vi "Warning Fault Tree View.vi"(0 "Model in":refnum<class "Model.lvclass">) -> ()   [LabVIEW 2016, in "M1M3SupportEUI_Views.lvlib"]
uses:
  M1M3SupportEUI_Views.lvlib
  Model/Model.lvclass
  M1M3 Support Events/M1M3 Support Events.lvclass/M1M3 Support Events.ctl
  M1M3 Support Events/M1M3 Support Events.lvclass
  EUI Events/EUI Events.lvclass
panel:
  in  "ClearAllErrors":bool
  in  "ClearOneError":bool
  in  "WarningTree":string(tree)
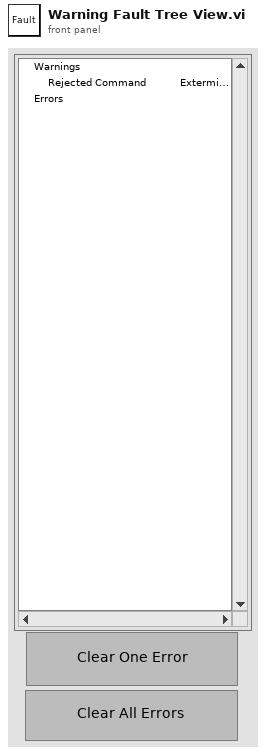
[diagram p1: front panel]
types:
  T1 = typedef "M1M3SupportEUI_TypeDefs.lvlib/M1M3 Support Events.ctl" = cluster{"Inclinometer  Data":refnum<user-event>, "IMS Data":refnum<user-event>, "SAL Connected":refnum<user-event>, "Accelerometer Data":refnum<user-event>, "OuterLoop Data":refnum<user-event>, "ErrorCode Event":refnum<user-event>, "InterlockStatus Event":refnum<user-event>, "InterlockWarning Event":refnum<user-event>, "Gyro Data":refnum<user-event>, "HP Actuator Info Event":refnum<user-event>, " FA Info Event":refnum<user-event>, "HP Monitor Info Event":refnum<user-event>, "FA Data":refnum<user-event>, "HP Actuator data":refnum<user-event>, "HP Monitor data":refnum<user-event>, "Air Supply Status Event":refnum<user-event>, "Air Supply Warning Event":refnum<user-event>, "Power Data":refnum<user-event>, "PID Data":refnum<user-event>, "PID Info Event":refnum<user-event>, "Power Status Event":refnum<user-event>, "Power Supply Status Event":refnum<user-event>, "Power Warning Event":refnum<user-event>, "Summary State Event":refnum<user-event>, "Detailed State Event":refnum<user-event>, "FA Force Warning Event":refnum<user-event>, "FA Warning Event":refnum<user-event>, "FA State Event":refnum<user-event>, "Applied AberrationForces Event":refnum<user-event>, "Applied Acceleration Forcces Event":refnum<user-event>, "Applied Azimuth Forces Event":refnum<user-event>, "Applied Active Optic Forces Event":refnum<user-event>, "Applied Balance Forces Event":refnum<user-event>, "Applied Cylinder Forces Event":refnum<user-event>, "Applied Elevation Forces Event":refnum<user-event>, "Applied Forces Event":refnum<user-event>, "Applied Offset Forces Event":refnum<user-event>, "Applied Static Forces Event":refnum<user-event>, "Applied Thermal Forces Event":refnum<user-event>, "Applied Velocity Forces Event":refnum<user-event>, "Rejected Aberration Force Event":refnum<user-event>, "Rejected Acceleration Forces Event":refnum<user-event>, "Rejected Active Optic Forces Event":refnum<user-event>, "Rejected Azimuth Forces Event":refnum<user-event>, "Rejected Balance Forces Event":refnum<user-event>, "Rejected Cylinder Forces Event":refnum<user-event>, "Rejected Elevation Forces Event":refnum<user-event>, "Rejected Forces Event":refnum<user-event>, "Rejected Offset Forces Event":refnum<user-event>, "Rejected Static Forces Event":refnum<user-event>, "Rejected Thermal Forces Event":refnum<user-event>, "Rejected Velocity Forces Event":refnum<user-event>, "Command Rejection Event":refnum<user-event>, "Setting Verions Event":refnum<user-event>, "Settings Applied Event":refnum<user-event>, "HP Actuator State Event":refnum<user-event>, "HP Actuator Warning Event":refnum<user-event>, "HP Monitor State Event":refnum<user-event>, "HP Monitor Warning Event":refnum<user-event>, "Accelerometer Warning Event":refnum<user-event>, "Applied Settings Match Start Event":refnum<user-event>, "Cell Light Status Event ":refnum<user-event>, "Cell Light Warning Event":refnum<user-event>, "Displacement Sensor Warning Event":refnum<user-event>, "Force Setpoint Warning Event":refnum<user-event>, "Gyro Warning Event ":refnum<user-event>, "ILC Warning Event ":refnum<user-event>, "Inclinometer Sensor Warning Event ":refnum<user-event>}
  T2 = enum16{"", "DetailedState_DetailedStates_DisabledState", "DetailedState_DetailedStates_EnabledState", "DetailedState_DetailedStates_FaultState", "DetailedState_DetailedStates_OfflineState", "DetailedState_DetailedStates_StandbyState", "DetailedState_DetailedStates_ParkedState", "DetailedState_DetailedStates_RaisingState", "DetailedState_DetailedStates_ActiveState", "DetailedState_DetailedStates_LoweringState", "DetailedState_DetailedStates_EngineeringState", "DetailedState_DetailedStates_ParkedEngineeringState", "DetailedState_DetailedStates_RaisingEngineeringState", "DetailedState_DetailedStates_ActiveEngineeringState", "DetailedState_DetailedStates_LoweringEngineeringState", "DetailedState_DetailedStates_LoweringFaultState", "DetailedState_DetailedStates_ProfileHardpointCorrectionState"}
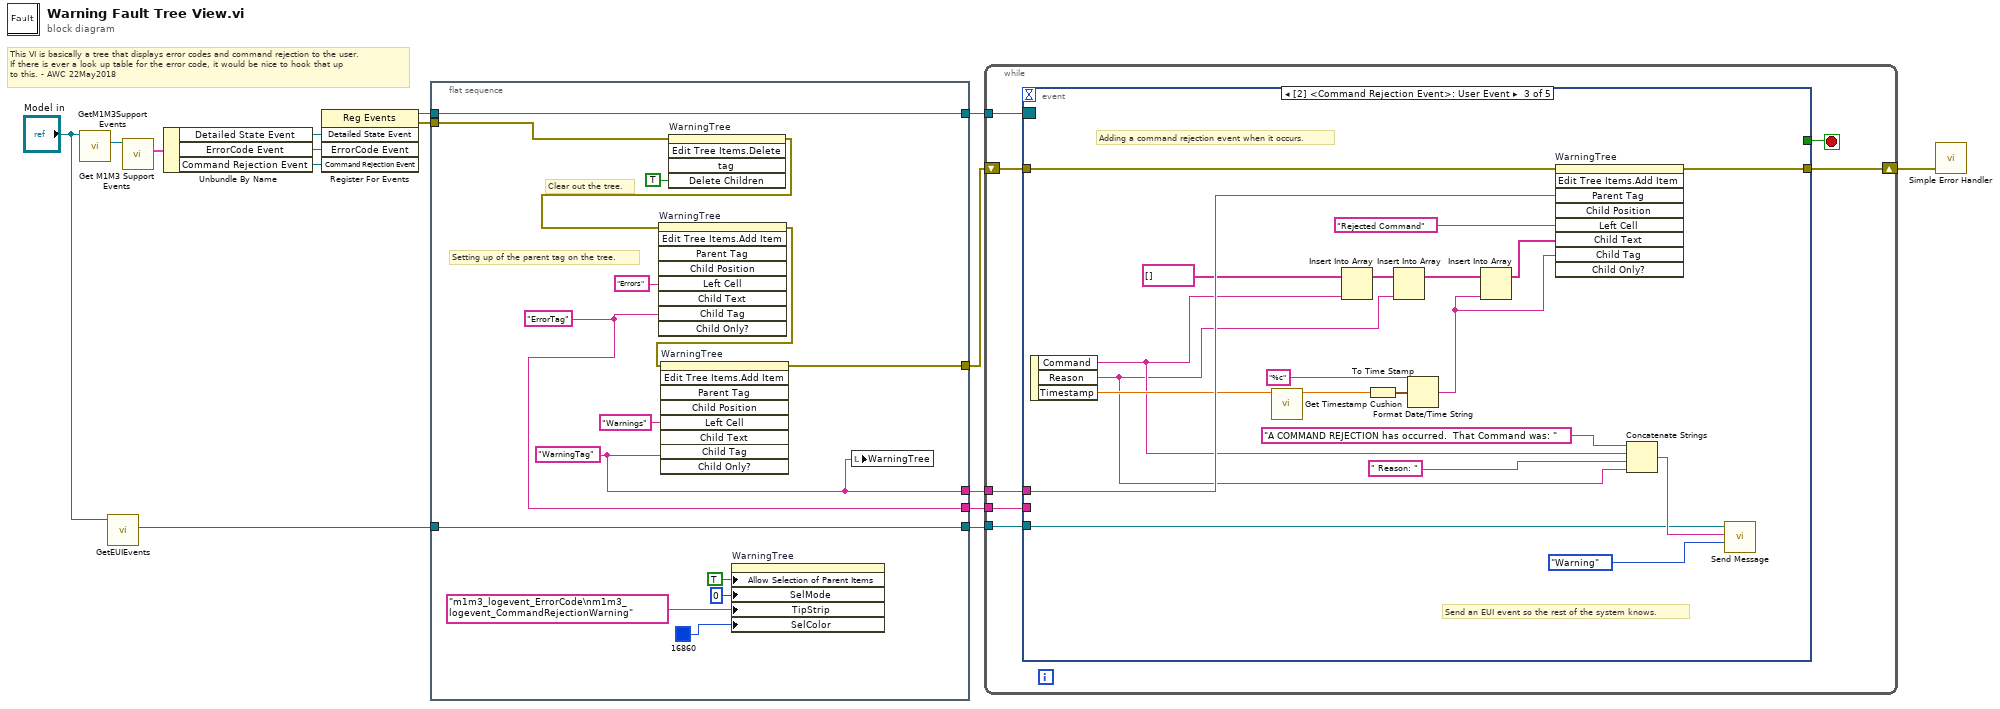
[diagram p0: block diagram]
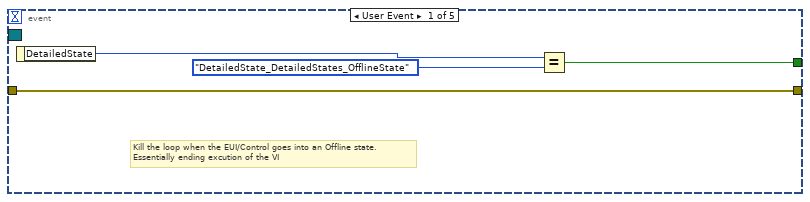
[diagram p2: hidden frame]
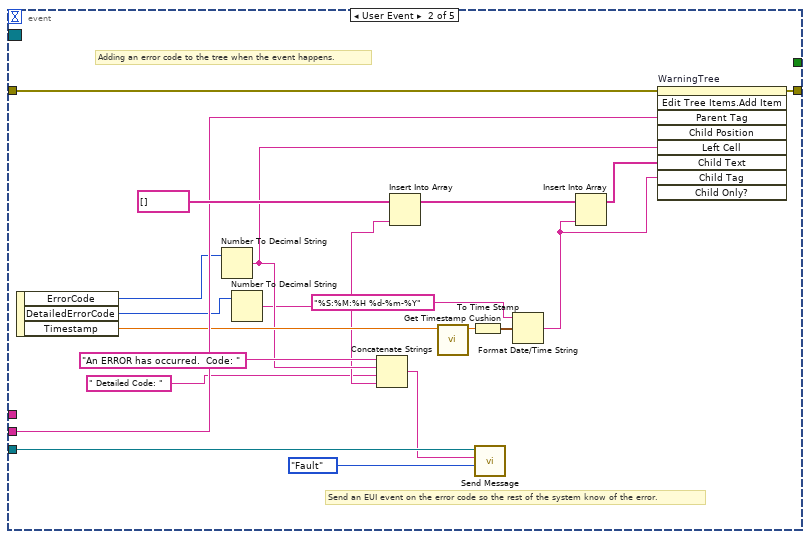
[diagram p3: hidden frame]
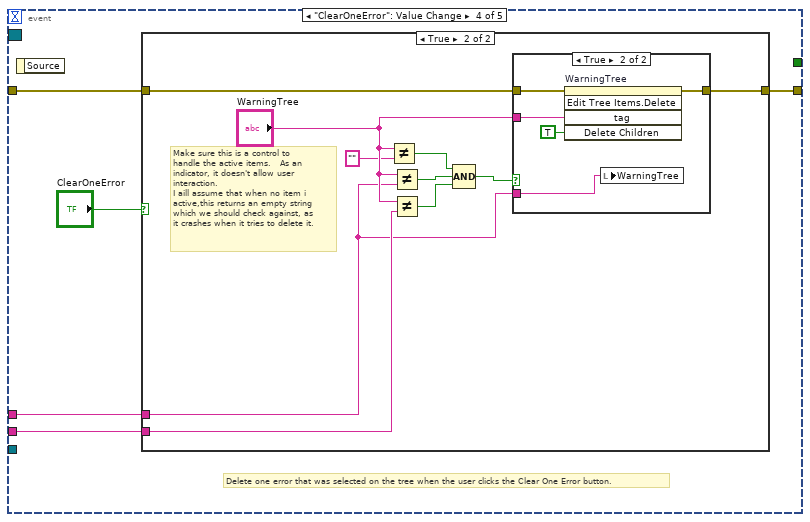
[diagram p4: hidden frame]
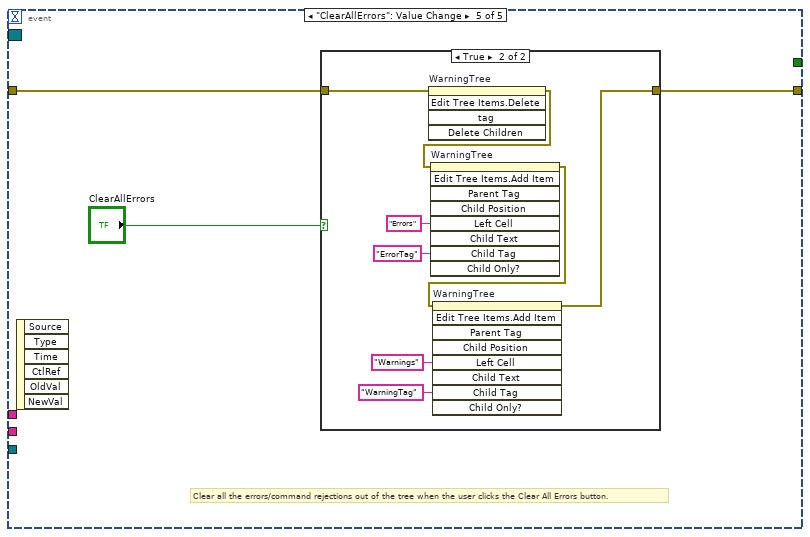
[diagram p7: hidden frame]
diagram:
  # "This VI is basically a tree that displays error codes and command rejection to the user.\nIf there is ever a look up table for the error code, it would be nice to hook that up\nto this. - AWC 22May2018"
  n1 = call "GetM1M3SupportEvents.vi"("Model in"="Model in") -> ("M1M3 Support Events out"=w11:refnum<class "M1M3 Support Events.lvclass">)  [unwired: 8 in, 2 out]
  n2 = call "GetEUIEvents.vi"("Model in"="Model in") -> ("EUI Events out"=w1:refnum<class "EUI Events.lvclass">)  [unwired: 8 in, 2 out]
  n3 = call "Get M1M3 Support Events.vi"("M1M3 Support Events in"=w11) -> ("M1M3 Support Events"=w12:T1)  [unwired: 9 in, 1 out]
  n4 = Unbundle By Name(w12) -> ("Detailed State Event"=w13:refnum<user-event>, "ErrorCode Event"=w14:refnum<user-event>, "Command Rejection Event"=w15:refnum<user-event>)
  n5 = register-events(w13, w14, w15) -> (reference out=w10:refnum<event-registration>, error out=w8:errorcluster)  [unwired: 2 in]
  n6 = flat-sequence {
    tunnel: w10 -> [w30]
    tunnel: [w30] -> w9
    tunnel: w8 -> [w18]
    tunnel: [w17] -> w7
    tunnel: [w16] -> w6
    tunnel: [w25] -> w5
    tunnel: w1 -> [w22]
    tunnel: [w22] -> w2
    frame #0 {
      w16 = "WarningTag" ("Child Tag")
      w25 = "ErrorTag" ("Child Tag")
      # "Clear out the tree."
      # "Setting up of the parent tag on the tree."
      n7 = invoke on="WarningTree" class="Tree (strict)" method="Edit Tree Items.Delete"(error in=w18, "Delete Children"=TRUE ("Delete Children?")) -> (error out=w29:errorcluster)  [unwired: 3 in, 4 out]
      n8 = invoke on="WarningTree" class="Tree (strict)" method="Edit Tree Items.Add Item"(error in=w29, "Left Cell"="Errors" ("Left Cell String"), "Child Tag"=w25) -> (error out=w27:errorcluster)  [unwired: 6 in, 8 out]
      n9 = invoke on="WarningTree" class="Tree (strict)" method="Edit Tree Items.Add Item"(error in=w27, "Left Cell"="Warnings" ("Left Cell String"), "Child Tag"=w16) -> (error out=w17:errorcluster)  [unwired: 6 in, 8 out]
      n10 = property on="WarningTree" class="Tree (strict)"("Allow Selection of Parent Items"=TRUE, "SelMode"=0 ("Selection Mode"), "TipStrip"="m1m3_logevent_ErrorCode\nm1m3_logevent_CommandRejectionWarning" ("Tip Strip"), "SelColor"=u32 16860) -> ()  [unwired: 2 in, 2 out]
      n11 = local write "WarningTree"(w16) -> ()
    }
  }
  n12 = while {
    tunnel: w9 -> [w37]
    shift-right: [w32] -> w4
    shift-left: w7 -> [w35]
    tunnel: w6 -> [w34]
    tunnel: w5 -> [w33]
    tunnel: w2 -> [w31]
    stop <- w36 stop-if-true
    n13 = event shown="[2] <Command Rejection Event>: User Event" {
      selector: w37 -> [_ _ _ _ _]
      dyn-events: _ -> [_ _ _ _ _]
      timeout: _ -> [_ _ _ _ _]
      tunnel: [w39 _ _ _ _] -> w36
      tunnel: w35 -> [w38 w56 w81 w85 w105]
      tunnel: w34 -> [_ _ w80 w83 _]
      tunnel: w33 -> [_ w55 _ w82 _]
      tunnel: [w38 w51 w70 w84 w104] -> w32
      tunnel: w31 -> [_ w49 w66 _ _]
      event User Event {
        # "Kill the loop when the EUI/Control goes into an Offline state.\nEssentially ending excution of the VI"
        n14 = event-data() -> ("DetailedState"=w41:T2)  [unwired: 1 in]
        n15 = Equal?(x=w41, y=T2."DetailedState_DetailedStates_OfflineState") -> (x = y?=w39:bool)
      }
      event User Event {
        # "Send an EUI event on the error code so the rest of the system know of the error."
        # "Adding an error code to the tree when the event happens."
        n16 = event-data() -> ("ErrorCode"=w53:i32, "DetailedErrorCode"=w52:i32, "Timestamp"=w54:dbl)  [unwired: 1 in]
        n17 = Number To Decimal String(number=w53) -> (decimal integer string=w47:string)  [unwired: 1 in]
        n18 = Number To Decimal String(number=w52) -> (decimal integer string=w46:string)  [unwired: 1 in]
        n19 = Concatenate Strings("An ERROR has occurred.  Code: " ("string"), w47, " Detailed Code: " ("string"), w46) -> (w44:string)
        n20 = Insert Into Array(array=string[] [], new element=w46) -> (w60:string[])  [unwired: 1 in]
        n21 = call "Get Timestamp Cushion.vi"("DoubleTimestampRepresentation"=w54) -> ("TimestampCushion"=w58:dbl)  [unwired: 10 in]
        n22 = To Time Stamp(1:w58) -> (0:w57:timestamp)
        n23 = call "Send Message.vi"("Priority"=enum16{"Message", "Warning", "Fault", ""}."Fault", "Message"=w44, "EUI Events in"=w49) -> ()  [unwired: 7 in, 2 out]
        n24 = Format Date/Time String(time format string (%c)="%S:%M:%H %d-%m-%Y", seconds (now)=w57) -> (date/time string=w42:string)  [unwired: 1 in]
        n25 = Insert Into Array(array=w60, new element=w42) -> (w59:string[])  [unwired: 1 in]
        n26 = invoke on="WarningTree" class="Tree (strict)" method="Edit Tree Items.Add Item"(error in=w56, "Parent Tag"=w55, "Left Cell"=w47, "Child Text"=w59, "Child Tag"=w42) -> (error out=w51:errorcluster)  [unwired: 4 in, 8 out]
      }
      event User Event {
        # "Send an EUI event so the rest of the system knows."
        # "Adding a command rejection event when it occurs."
        n27 = event-data() -> ("Command"=w65:string, "Reason"=w64:string, "Timestamp"=w72:dbl)  [unwired: 1 in]
        n28 = call "Get Timestamp Cushion.vi"("DoubleTimestampRepresentation"=w72) -> ("TimestampCushion"=w74:dbl)  [unwired: 10 in]
        n29 = Insert Into Array(array=string[] [], new element=w65) -> (w77:string[])  [unwired: 1 in]
        n30 = To Time Stamp(1:w74) -> (0:w73:timestamp)
        n31 = Insert Into Array(array=w77, new element=w64) -> (w76:string[])  [unwired: 1 in]
        n32 = Format Date/Time String(time format string (%c)="%c", seconds (now)=w73) -> (date/time string=w62:string)  [unwired: 1 in]
        n33 = Insert Into Array(array=w76, new element=w62) -> (w75:string[])  [unwired: 1 in]
        n34 = invoke on="WarningTree" class="Tree (strict)" method="Edit Tree Items.Add Item"(error in=w81, "Parent Tag"=w80, "Left Cell"="Rejected Command" ("Left Cell String"), "Child Text"=w75, "Child Tag"=w62) -> (error out=w70:errorcluster)  [unwired: 4 in, 8 out]
        n35 = Concatenate Strings("A COMMAND REJECTION has occurred.  That Command was: " ("string"), w65, " Reason: " ("string"), w64) -> (w67:string)
        n36 = call "Send Message.vi"("Priority"=enum16{"Message", "Warning", "Fault", ""}."Warning", "Message"=w67, "EUI Events in"=w66) -> ()  [unwired: 7 in, 2 out]
      }
      event "ClearOneError": Value Change {
        # "Delete one error that was selected on the tree when the user clicks the Clear One Error button."
        n37 = event-data() -> ()  [unwired: 1 in, 1 out]
        n38 = case shown="True" "ClearOneError" {
          tunnel: w85 -> [w87 w92]
          tunnel: [w87 w97] -> w84
          tunnel: w83 -> [_ w88]
          tunnel: w82 -> [_ w96]
          frame False {
          }
          frame True {
            # "Make sure this is a control to \nhandle the active items.   As an \nindicator, it doesn't allow user\ninteraction.\nI aill assume that when no item i\nactive,this returns an empty string\nwhich we should check against, as\nit crashes when it tries to delete it."
            n39 = Not Equal?(x="WarningTree", y="") -> (x != y?=w91:bool)
            n40 = Not Equal?(x="WarningTree", y=w88) -> (x != y?=w94:bool)
            n41 = Not Equal?(x="WarningTree", y=w96) -> (x != y?=w95:bool)
            n42 = Compound Arithmetic op=AND(w91, w94, w95) -> (w93:bool)
            n43 = case shown="True" w93 {
              tunnel: w92 -> [w98 w103]
              tunnel: "WarningTree" -> [_ w102]
              tunnel: [w98 w100] -> w97
              tunnel: w88 -> [_ w99]
              frame False {
              }
              frame True {
                n44 = invoke on="WarningTree" class="Tree (strict)" method="Edit Tree Items.Delete"(error in=w103, "tag"=w102, "Delete Children"=TRUE ("Delete Children?")) -> (error out=w100:errorcluster)  [unwired: 2 in, 4 out]
                n45 = local write "WarningTree"(w99) -> ()
              }
            }
          }
        }
      }
      event "ClearAllErrors": Value Change {
        # "Clear all the errors/command rejections out of the tree when the user clicks the Clear All Errors button."
        n46 = event-data() -> ()  [unwired: 1 in, 6 out]
        n47 = case shown="True" "ClearAllErrors" {
          tunnel: w105 -> [w107 w115]
          tunnel: [w107 w108] -> w104
          frame False {
          }
          frame True {
            n48 = invoke on="WarningTree" class="Tree (strict)" method="Edit Tree Items.Delete"(error in=w115) -> (error out=w109:errorcluster)  [unwired: 4 in, 4 out]
            n49 = invoke on="WarningTree" class="Tree (strict)" method="Edit Tree Items.Add Item"(error in=w109, "Left Cell"="Errors" ("Left Cell String"), "Child Tag"="ErrorTag") -> (error out=w112:errorcluster)  [unwired: 6 in, 8 out]
            n50 = invoke on="WarningTree" class="Tree (strict)" method="Edit Tree Items.Add Item"(error in=w112, "Left Cell"="Warnings" ("Left Cell String"), "Child Tag"="WarningTag") -> (error out=w108:errorcluster)  [unwired: 6 in, 8 out]
          }
        }
      }
    }
  }
  n51 = call <vilib>:"Simple Error Handler.vi"("error in (no error)"=w4) -> ()  [unwired: 4 in, 5 out]
